vi "Vision Research Phantom Series PhCon PhDeleteCine.vi"(0 "CN in":u32=1, 1 "Cine":i32, 5 "Error In (no error)":errorcluster) -> (14 "CN out":u32=1, 19 "Error Out":errorcluster)   [LabVIEW 2013, in "VRI.lvlib"]
doc: "PhCon dll\n\nPhDeleteCine\nHRESULT PhDeleteCine(UINT CN, int Cine);\n\nParameters Description\nCN (in) Camera number.\nCine (in) Cine number.\nReturn HRESULT (0=Ok)\nComments Delete the specified cine. A new recording may use the\n parameters and the space of the new cine.\n\nWritten by:\nBLOOMY CONTROLS, INC\nWINDSOR, CT 06095, USA\n860-298-9925\nwww.bloomy.com\nV1.0.0\nMay, 2004"
uses:
  VRI.lvlib
  Phantom DLLs/PhCon.Dll
panel:
  # "For instructions on the use of this VI, press Ctrl+H to display the help window and move the mouse over the icon, controls, and indicators"
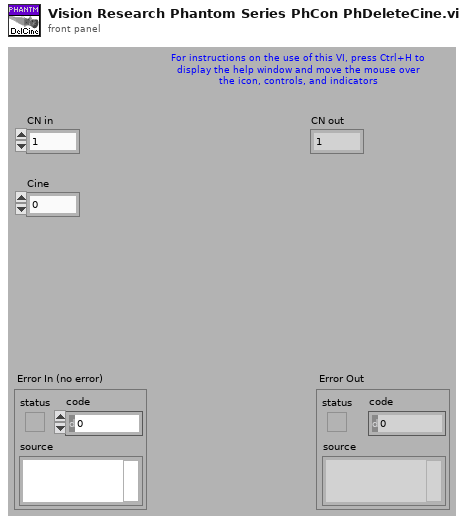
[diagram p1: front panel]
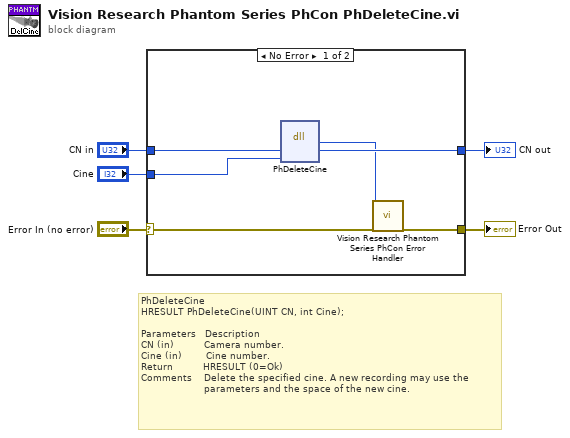
[diagram p0: block diagram]
diagram:
  # "PhDeleteCine\nHRESULT PhDeleteCine(UINT CN, int Cine);\n\nParameters   Description\nCN (in)          Camera number.\nCine (in)        Cine number.\nReturn          HRESULT (0=Ok)\nComments    Delete the specified cine. A new recording may use the\n                     parameters and the space of the new cine."
  n1 = case shown="No Error" "Error In (no error)" {
    selector: "Error In (no error)" -> [w11 w13]
    tunnel: [w10 w13] -> w4
    tunnel: "CN in" -> [w9 w12]
    tunnel: [w8 w12] -> w2
    tunnel: "Cine" -> [w7 _]
    frame No Error {
      n2 = dll-call lib="C:/Projects/SDK/64-bit/Vision Research Phantom Series Labview Driver/Phantom DLLs/PhCon.dll" fn="PhDeleteCine"("CN"=w9, "Cine"=w7) -> ("HRESULT"=w6:i32, "CN"=w8:u32)  [unwired: 4 in, 2 out]
      n3 = call "Vision Research Phantom Series PhCon Error Handler.vi"("ErrNo"=w6, "Error In (no error)"=w11) -> ("Error Out"=w10:errorcluster)  [unwired: 17 out]
    }
    frame Error {
    }
  }
  "Error Out" <- w4
  "CN out" <- w2
